vi "Send_Classification_Frame.vi"(5 "error in (no error)":errorcluster, 6 "rt fifo single":refnum<k33>, 8 "Pre-Partition":sgl[][](array[numeric])) -> (0 "error out":errorcluster, 3 "Sended frame":dbl[](array[numeric]))   [LabVIEW 2020]
panel:
  out "Average Pupil":dbl
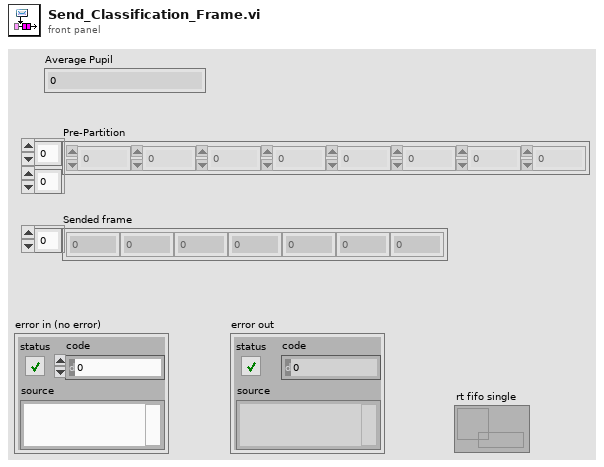
[diagram p1: front panel]
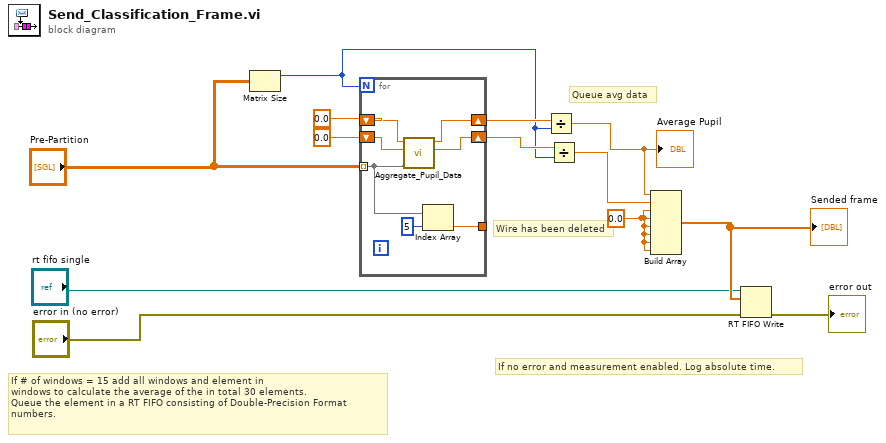
[diagram p0: block diagram]
diagram:
  w1 = 0.0 ("element")
  # "Wire has been deleted"
  # "Queue avg data"
  # "If no error and measurement enabled. Log absolute time."
  # "If # of windows = 15 add all windows and element in \nwindows to calculate the average of the in total 30 elements. \nQueue the element in a RT FIFO consisting of Double-Precision Format \nnumbers."
  n1 = Matrix Size(0:"Pre-Partition") -> (1:w5:i32)  [unwired: 1 out]
  n2 = for {
    N: w5 -> [_]
    shift-right: [w18] -> w12
    shift-left: 0.0 -> [w20]
    shift-right: [w17] -> w10
    shift-left: 0.0 -> [w19]
    tunnel: [w15] -> _
    tunnel: "Pre-Partition" -> [w14] mode=indexing
    n3 = call "Aggregate_Pupil_Data.vi"("Subarray"=w14, "Partial Sum R"=w19, "Partial Sum  L"=w20) -> ("Sum R"=w17:dbl, "Sum L"=w18:dbl)  [unwired: 7 in]
    n4 = Index Array(array=w14, index=5) -> (element=w15:sgl)
  }
  n5 = Divide(x=w12, y=w5) -> (x/y=w3:dbl)
  "Average Pupil" <- w3
  n6 = Divide(x=w10, y=w5) -> (x/y=w2:dbl)
  n7 = Build Array(w3, w2, w1, w1, w1, w1, w1, w1) -> (w9:dbl[])
  "Sended frame" <- w9
  n8 = RT FIFO Write(0:"rt fifo single", 1:w9, 3:"error in (no error)") -> (11:→"error out":errorcluster)  [unwired: 2 in, 3 out]
